vi "Z900_navX_SERIAL_Read.vi"(8 "error in (no error)":errorcluster, 10 "Registry":u8[](array[numeric]), 11 "Interface TypeDefs":T1 {"I2CDevRef"."Device Address" format="%.0x"}) -> (0 "error out":errorcluster, 1 "Valid":bool, 2 "Registry":u8[](array[numeric]), 3 "Interface TypeDefs":T1 {"I2CDevRef"."Device Address" format="%.0x"})   [LabVIEW 2015, in "navX Library v2.lvlib"]
uses:
  navX Library v2.lvlib
  _TypeDefs/Z900_navX_InterfaceTypeDef.ctl
  <vilib>/Rock Robotics/WPI/SerialPort/WPI_SerialPortRef.ctl
  <vilib>/Rock Robotics/WPI/I2C/WPI_I2CDevRef.ctl
  <vilib>/Rock Robotics/SystemInterfaces/i2clib/i2c_bus.ctl
  <vilib>/Rock Robotics/WPI/SPI/WPI_SPIDevRef.ctl
  <vilib>/Rock Robotics/SystemInterfaces/spilib/spi_bus.ctl
  Z900_navX_SERIAL_ValidatePacketChecksum.vi
  Z900_navX_SERIAL_ValidatePacketTermination.vi
  _Util/Encode Protocol/Z900_navX_Util_EncodeProtocol_SignedHundredths.vi
  _Util/Encode Protocol/Z900_navX_Util_EncodeProtocol_UnsignedHundredths.vi
  _Util/Encode Protocol/Z900_navX_Util_EncodeProtocol_UInt16.vi
  _Util/Encode Protocol/Z900_navX_Util_EncodeProtocol_Int16.vi
  _Util/Z900_navX_Util_BigEndian_to_LittleEndian.vi
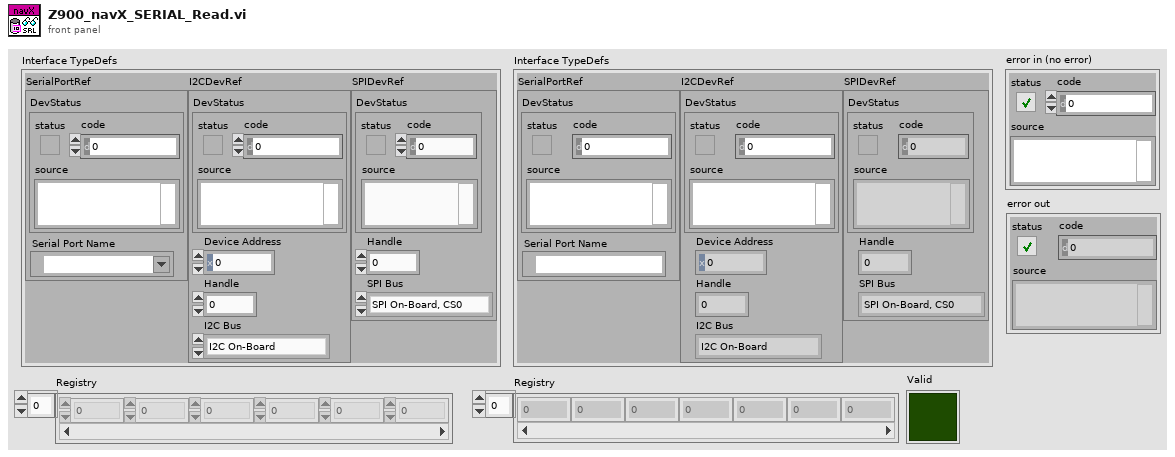
[diagram p1: front panel]
types:
  T1 = typedef "navX Library v2.lvlib/Z900_navX_InterfaceTypeDef.ctl" = cluster{"SerialPortRef":T2, "I2CDevRef":T3, "SPIDevRef":T5}
  T2 = typedef "WPI_SerialPortRef.ctl" = cluster{"DevStatus":errorcluster, "Serial Port Name":refnum<visa-resource-name>}
  T3 = typedef "WPI_I2CDevRef.ctl" = cluster{"DevStatus":errorcluster, "Device Address":u8, "Handle":i32, "I2C Bus":T4}
  T4 = typedef "i2c_bus.ctl" = enum16{"I2C On-Board", "I2C MXP", "Invalid"}
  T5 = typedef "WPI_SPIDevRef.ctl" = cluster{"DevStatus":errorcluster, "Handle":i32, "SPI Bus":T6}
  T6 = typedef "spi_bus.ctl" = enum16{"SPI On-Board, CS0", "SPI On-Board, CS1", "SPI On-Board, CS2", "SPI On-Board, CS3", "SPI MXP", "Invalid"}
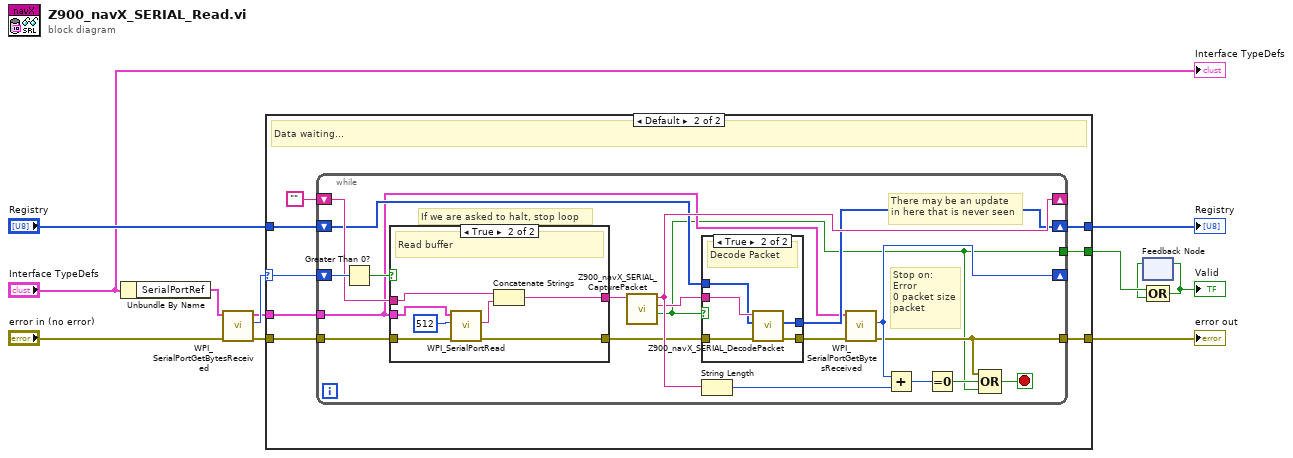
[diagram p0: block diagram]
diagram:
  n1 = Unbundle By Name("Interface TypeDefs") -> ("SerialPortRef"=w12:T2)
  n2 = call <vilib>:"WPI_SerialPortGetBytesReceived.vi"("error in (no error)"="error in (no error)", "SerialPortRef"=w12) -> ("error out"=w10:errorcluster, "Bytes at Port"=w11:u32, "SerialPortRef"=w9:T2)  [unwired: 7 in]
  n3 = case shown="Default" w11 {
    selector: w11 -> [_ w17]
    tunnel: [w14 w22] -> w7
    tunnel: "Registry" -> [w14 w21]
    tunnel: w9 -> [_ w19]
    tunnel: w10 -> [w13 w18]
    tunnel: [w13 w16] -> w5
    tunnel: [_ w15] -> w3
    frame 0 {
    }
    frame Default {
      # "Data waiting..."
      n4 = while {
        shift-right: [w29] -> w22
        shift-left: w21 -> [w34]
        shift-right: [w37] -> _
        shift-left: w17 -> [w41]
        shift-right: [w36] -> _
        shift-left: "" -> [w40]
        tunnel: w19 -> [w24]
        tunnel: w18 -> [w39]
        tunnel: [w27] -> w16
        tunnel: [w23] -> w15
        stop <- w28 stop-if-true
        # "Stop on:\nError\n0 packet size\npacket"
        # "There may be an update\nin here that is never seen"
        # "If we are asked to halt, stop loop"
        n5 = Greater Than 0?(x=w41) -> (x > 0?=w30:bool)
        n6 = case shown="True" w30 {
          tunnel: w40 -> [w50 w57]
          tunnel: w24 -> [_ w56]
          tunnel: w39 -> [w49 w53]
          tunnel: [w50 w52] -> w38
          tunnel: [w49 w51] -> w33
          frame False {
            # "Pass existing buffer"
          }
          frame True {
            # "Read buffer"
            n7 = call <vilib>:"WPI_SerialPortRead.vi"("error in (no error)"=w53, "Num Bytes to Read"=u32 512, "SerialPortRef"=w56) -> ("error out"=w51:errorcluster, "Buffer"=w55:string)  [unwired: 6 in, 1 out]
            n8 = Concatenate Strings(w57, w55) -> (w52:string)
          }
        }
        n9 = call "Z900_navX_SERIAL_CapturePacket.vi"("Buffer"=w38) -> ("Packet Located"=w23:bool, "Packet"=w35:string, "Buffer"=w36:string)  [unwired: 7 in, 1 out]
        n10 = case shown="True" w23 {
          tunnel: w35 -> [_ w48]
          tunnel: [w43 w46] -> w29
          tunnel: w34 -> [w43 w47]
          tunnel: w33 -> [w42 w45]
          tunnel: [w42 w44] -> w32
          frame False {
            # "No Packet"
          }
          frame True {
            # "Decode Packet"
            n11 = call "Z900_navX_SERIAL_DecodePacket.vi"("error in (no error)"=w45, "Data"=w47, "Packet"=w48) -> ("error out"=w44:errorcluster, "Data"=w46:u8[])  [unwired: 6 in, 1 out]
          }
        }
        n12 = String Length(string=w36) -> (length=w25:i32)
        n13 = call <vilib>:"WPI_SerialPortGetBytesReceived.vi"("error in (no error)"=w32, "SerialPortRef"=w24) -> ("error out"=w27:errorcluster, "Bytes at Port"=w37:u32)  [unwired: 7 in, 1 out]
        n14 = Add(x=w37, y=w25) -> (x+y=w26:u32)
        n15 = Equal To 0?(x=w26) -> (x = 0?=w31:bool)
        n16 = Compound Arithmetic op=OR(w27, w31, w23) -> (w28:bool)
      }
    }
  }
  "Registry" <- w7
  "error out" <- w5
  n17 = feedback #1() -> (w2:bool)  [unwired: 1 in]
  n18 = Compound Arithmetic op=OR(w3, w2) -> (w1:bool)
  "Valid" <- w1
  n19 = feedback-in #1(w1) -> ()
  "Interface TypeDefs" <- "Interface TypeDefs"
